vi "read_and_write.vi"(4 "additional waiting time":u32, 5 "waypoint version":bool, 6 "semaphore":T1, 7 "Motor Adress":T2(ring)=enum."3", 8 "error in (no error)":errorcluster, 9 "Command":string, 10 "value":i32=123456, 11 "VISA ressource in":refnum<visa-resource-name>="COM1") -> (0 "error out":errorcluster={"status"=FALSE, "code"=1073676294, "source"="VISA Read in write_read.vi"}, 1 "Answer":string, 2 "Log File (global)":string, 3 "VISA ressource out":refnum<visa-resource-name>)   [LabVIEW 2013]
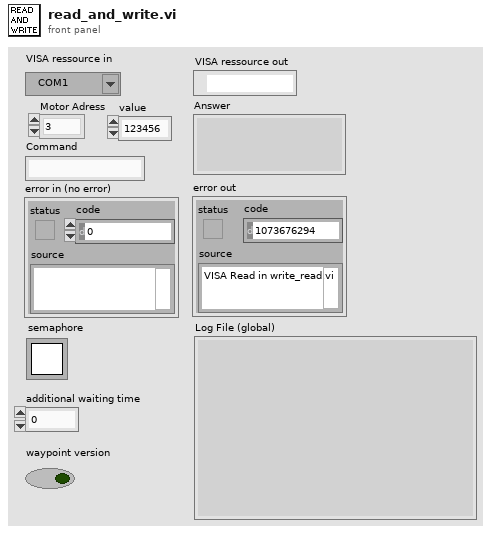
[diagram p1: front panel]
types:
  T1 = typedef "Semaphore RefNum" = refnum<k1>
  T2 = enum16{"All", "1", "2", "3", "4", "5", "6", "7", "8"}
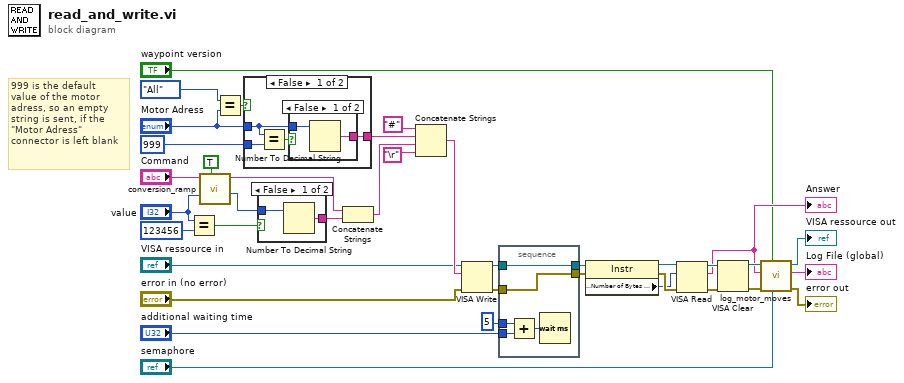
[diagram p0: block diagram]
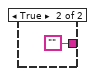
[diagram p2: hidden frame]
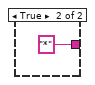
[diagram p3: hidden frame]
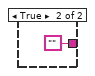
[diagram p4: hidden frame]
diagram:
  # "999 is the default\nvalue of the motor\nadress, so an empty\nstring is sent, if the\n\"Motor Adress\"\nconnector is left blank"
  n1 = Equal?(x="value", y=123456 ("x")) -> (x = y?=w28:bool)
  n2 = call "conversion_ramp.vi"("From Hz/ms to Driver"=TRUE, "Value"="value", "Command"="Command") -> ("Value out"=w4:i32, "String"=w8:string)  [unwired: 7 in]
  n3 = Equal?(x=T2."All", y="Motor Adress") -> (x = y?=w24:bool)
  n4 = case shown="False" w24 {
    tunnel: u16 999 ("x") -> [w41 _]
    tunnel: "Motor Adress" -> [w40 _]
    tunnel: [w39 "*"] -> w23
    frame False {
      n5 = Equal?(x=w40, y=w41) -> (x = y?=w42:bool)
      n6 = case shown="False" w42 {
        tunnel: [w44 ""] -> w39
        tunnel: w40 -> [w43 _]
        frame False {
          n7 = Number To Decimal String(number=w43) -> (decimal integer string=w44:string)  [unwired: 1 in]
        }
        frame True {
        }
      }
    }
    frame True {
    }
  }
  n8 = case shown="False" w28 {
    tunnel: [w48 ""] -> w29
    tunnel: w4 -> [w47 _]
    frame False {
      n9 = Number To Decimal String(number=w47) -> (decimal integer string=w48:string)  [unwired: 1 in]
    }
    frame True {
    }
  }
  n10 = Concatenate Strings(w8, w29) -> (w30:string)
  n11 = Concatenate Strings("#" ("staticText"), w23, w30, "\r") -> (w36:string)
  n12 = VISA Write(VISA resource name="VISA ressource in", write buffer=w36, error in (no error)="error in (no error)") -> (VISA resource name out=w22:refnum<visa-resource-name>, error out=w20:errorcluster)  [unwired: 1 out]
  n13 = stacked-sequence {
    tunnel: w22 -> [w54]
    tunnel: [w54] -> w21
    tunnel: w20 -> [w53]
    tunnel: [w53] -> w19
    tunnel: "additional waiting time" -> [w51]
    tunnel: u32 5 ("milliseconds to wait") -> [w50]
    frame #0 {
      n14 = Add(x=w50, y=w51) -> (x+y=w52:u32)
      n15 = Wait (ms)(milliseconds to wait=w52) -> ()  [unwired: 1 out]
    }
  }
  n16 = property class="Instr"(reference=w21, error in=w19) -> (reference out=w32:refnum<visa-resource-name>, error out=w33:errorcluster, "Serial Settings:Number of Bytes at Serial Port"=w31:u32)
  n17 = VISA Read(VISA resource name=w32, byte count=w31, error in (no error)=w33) -> (VISA resource name out=w35:refnum<visa-resource-name>, read buffer=w12:string, error out=w34:errorcluster)  [unwired: 1 out]
  "Answer" <- w12
  n18 = VISA Clear(VISA resource name=w35, error in (no error)=w34) -> (VISA resource name out=w15:refnum<visa-resource-name>, error out=w16:errorcluster)
  n19 = call "log_motor_moves.vi"("semaphore"="semaphore", "waypoint version"="waypoint version", "error in (no error)"=w16, "Answer"=w12, "VISA resource name"=w15) -> ("error out"=→"error out":errorcluster, "Log File"=→"Log File (global)":string, "VISA resource name out"=→"VISA ressource out":refnum<visa-resource-name>)  [unwired: 4 in]
